vi "Import - Main.vi"(6 "New CD?":bool, 7 "Device Item Ref in":T19 format="%.0x", 8 "error in (no error)":errorcluster, 11 "Import/Export Data":T1 {"Tx Packets"."Tx Packet Data"."threadOptions"."pclDecimation" max=16 step=1; "Tx Packets"."Tx Packet Data"."threadOptions"."loopPeriod" max=16 step=1; "Tx Packets"."Tx Packet Data"."threadOptions"."targetPriority" min=-2 max=16 step=1; "Tx Packets"."Tx Packet Data"."threadOptions"."targetProcessor" min=-2 max=16 step=1; "Tx Packets"."Tx Packet Data"."Endianness" items=["big-endian"=0, "little-endian"=2]; "Rx Packets"."Rx Packet Data"."targetPriority" min=-2 max=16 step=1; "Rx Packets"."Rx Packet Data"."targetProcessor" min=-2 max=16 step=1; "Rx Packets"."Rx Packet Data"."Endianness" items=["big-endian"=0, "little-endian"=2]}) -> (0 "error out":errorcluster)   [LabVIEW 2019, in "UDP-Custom-Device System Explorer.lvlib"]
uses:
  UDP-Custom-Device System Explorer.lvlib
  <vilib>/NI VeriStand/Custom Device API/Custom Device Item Ref.ctl
  Types/XML - New/ImpExp - Data.ctl
  Types/XML - New/ImpExp - Main Data.ctl
  <vilib>/NI VeriStand/Custom Device API/Custom Device Item Info.ctl
  Types/XML - New/ImpExp - Rx Packets Data.ctl
  Types/XML - New/ImpExp - Rx Packet Data.ctl
  Shared/Types/Shared - Channel Data Type.ctl
  Shared/Types/Shared - Buffered.PacketInfo.ctl
  Shared/Types/Shared - Pointer Encoding.ctl
  Shared/Types/Shared - Receive Buffer Options.ctl
  Shared/Types/Shared - Transmit Buffer Options.ctl
  Shared/Types/Shared - New Data Options.ctl
  Shared/Types/Shared - Thread Management.ctl
  Types/XML - New/ImpExp - Tx Packets Data.ctl
  Types/XML - New/ImpExp - Tx Packet Data.ctl
  Shared/Types/Shared - Transmit Flag Options.ctl
  Shared/Types/Shared - Transmit Echo Options.ctl
  Types/Threading/Thread Configuration.ctl
  Types/Threading/Thread Sync Reference.ctl
  Property Accessors/Main Accessors.lvlib
  <vilib>/NI VeriStand/Custom Device API/Custom Device API.lvlib
  <vilib>/NI VeriStand/Custom Device Tools/Custom Device Utility Library/Custom Device Utility Library.lvlib
  Shared/UDP-Custom-Device Shared.lvlib
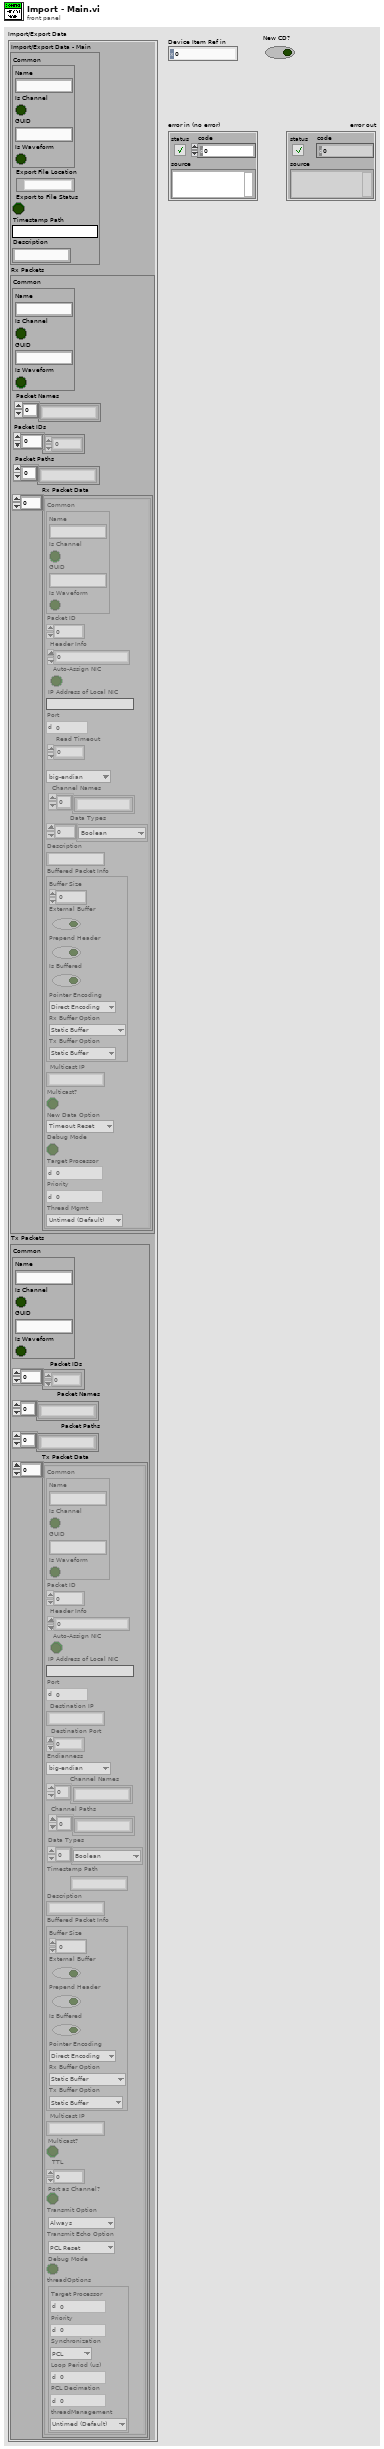
[diagram p1: front panel]
types:
  T1 = typedef "UDP-Custom-Device System Explorer.lvlib/ImpExp - Data.ctl" = cluster{"Import/Export Data - Main":T2, "Rx Packets":T4, "Tx Packets":T13}
  T2 = typedef "UDP-Custom-Device System Explorer.lvlib/ImpExp - Main Data.ctl" = cluster{"Common":T3, "Export File Location":path, "Export to File Status":bool, "Timestamp Path":string, "Description":string}
  T3 = typedef "Custom Device API.lvlib/Custom Device Item Info.ctl" = cluster{"Name":string, "Is Channel":bool, "GUID":string, "Is Waveform":bool}
  T4 = typedef "UDP-Custom-Device System Explorer.lvlib/ImpExp - Rx Packets Data.ctl" = cluster{"Common":T3, "Packet Names":string[], "Packet IDs":i32[], "Packet Paths":string[], "Rx Packet Data":T5[]}
  T5 = typedef "UDP-Custom-Device System Explorer.lvlib/ImpExp - Rx Packet Data.ctl" = cluster{"Common":T3, "Packet ID":i32, "Header Info":u32, "Auto-Assign NIC":bool, "IP Address of Local NIC":string, "Port":u16, "Read Timeout":i32, "Endianness":u16, "Channel Names":string[], "Data Types":T6[], "Description":string, "Buffered Packet Info":T7, "Multicast IP":string, "Multicast?":bool, "New Data Option":T11, "Debug Mode":bool, "targetProcessor":i8, "targetPriority":i16, "Thread Mgmt":T12}
  T6 = typedef "UDP-Custom-Device Shared.lvlib/Shared - Channel Data Type.ctl" = enum16{"Boolean", "Single", "Double", "I8", "I16", "I32", "I64", "U8", "U16", "U32", "U64"}
  T7 = typedef "UDP-Custom-Device Shared.lvlib/Shared - Buffered.PacketInfo.ctl" = cluster{"Buffer Size":i32, "External Buffer":bool, "Prepend Header":bool, "Is Buffered":bool, "Pointer Encoding":T8, "Rx Buffer Option":T9, "Tx Buffer Option":T10}
  T8 = typedef "UDP-Custom-Device Shared.lvlib/Shared - Pointer Encoding.ctl" = enum16{"Direct Encoding", "Conversion Encoding"}
  T9 = typedef "UDP-Custom-Device Shared.lvlib/Shared - Receive Buffer Options.ctl" = enum16{"Static Buffer", "Circular Buffer", "Circular Buffer + Size", "Internal Cache", "Internal Cache + Size", "Ping Pong", "Ping Pong + Size"}
  T10 = typedef "UDP-Custom-Device Shared.lvlib/Shared - Transmit Buffer Options.ctl" = enum16{"Static Buffer", "FIFO Buffer", "FIFO Buffer + Port"}
  T11 = typedef "UDP-Custom-Device Shared.lvlib/Shared - New Data Options.ctl" = enum16{"Timeout Reset", "Counter"}
  T12 = typedef "UDP-Custom-Device Shared.lvlib/Shared - Thread Management.ctl" = enum16{"Untimed (Default)", "Timed (High Priority)"}
  T13 = typedef "UDP-Custom-Device System Explorer.lvlib/ImpExp - Tx Packets Data.ctl" = cluster{"Common":T3, "Packet IDs":i32[], "Packet Names":string[], "Packet Paths":string[], "Tx Packet Data":T14[]}
  T14 = typedef "UDP-Custom-Device System Explorer.lvlib/ImpExp - Tx Packet Data.ctl" = cluster{"Common":T3, "Packet ID":i32, "Header Info":u32, "Auto-Assign NIC":bool, "IP Address of Local NIC":string, "Port":u16, "Destination IP":string, "Destination Port":u16, "Endianness":u16, "Channel Names":string[], "Channel Paths":string[], "Data Types":T6[], "Timestamp Path":string, "Description":string, "Buffered Packet Info":T7, "Multicast IP":string, "Multicast?":bool, "TTL":u16, "Port as Channel?":bool, "Transmit Option":T15, "Transmit Echo Option":T16, "Debug Mode":bool, "threadOptions":T17}
  T15 = typedef "UDP-Custom-Device Shared.lvlib/Shared - Transmit Flag Options.ctl" = enum16{"Always", "One-Shot", "Toggle"}
  T16 = typedef "UDP-Custom-Device Shared.lvlib/Shared - Transmit Echo Options.ctl" = enum16{"PCL Reset", "Counter", "Mirror"}
  T17 = typedef "UDP-Custom-Device System Explorer.lvlib/Thread Configuration.ctl" = cluster{"targetProcessor":i8, "targetPriority":i16, "Synchronization":T18, "loopPeriod":u32, "pclDecimation":u16, "threadManagement":T12}
  T18 = typedef "UDP-Custom-Device System Explorer.lvlib/Thread Sync Reference.ctl" = enum16{"PCL", "Async"}
  T19 = typedef "Custom Device API.lvlib/Custom Device Item Ref.ctl" = u64
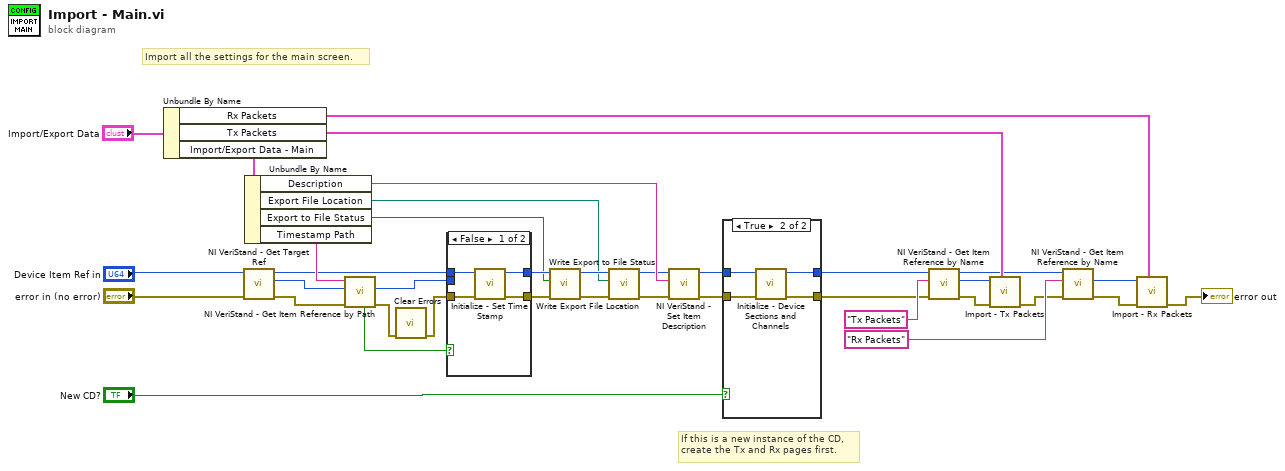
[diagram p0: block diagram]
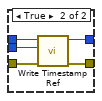
[diagram p2: hidden frame]
diagram:
  # "If this is a new instance of the CD,\ncreate the Tx and Rx pages first."
  # "Import all the settings for the main screen."
  n1 = Unbundle By Name("Import/Export Data") -> ("Rx Packets"=w17:T4, "Tx Packets"=w16:T13, "Import/Export Data - Main"=w36:T2)
  n2 = call <vilib>:"NI VeriStand - Get Target Ref.vi"("error in"="error in (no error)", "Item Ref in"="Device Item Ref in") -> ("error out"=w31:errorcluster, "Target Ref"=w33:T19, "Item Ref out"=w30:T19)  [unwired: 6 in, 1 out]
  n3 = Unbundle By Name(w36) -> ("Description"=w20:string, "Export File Location"=w21:path, "Export to File Status"=w22:bool, "Timestamp Path"=w35:string)
  n4 = call <vilib>:"NI VeriStand - Get Item Reference by Path.vi"("error in (no error)"=w31, "Root Ref"=w33, "Item Path in"=w35) -> ("error out"=w28:errorcluster, "Item Ref"=w29:T19, "Found"=w1:bool)  [unwired: 5 in, 1 out]
  n5 = call <vilib>:"Clear Errors.vi"("error in (no error)"=w28) -> ("error out"=w27:errorcluster)  [unwired: 5 in, 1 out]
  n6 = case shown="False" w1 {
    tunnel: w30 -> [w41 w46]
    tunnel: w29 -> [_ w45]
    tunnel: w27 -> [w39 w44]
    tunnel: [w40 w43] -> w26
    tunnel: [w38 w42] -> w25
    frame False {
      n7 = call "Initialize - Set Time Stamp.vi"("error in (no error)"=w39, "Device Item Ref in"=w41) -> ("error out"=w38:errorcluster, "Device Item Ref out"=w40:T19)  [unwired: 7 in, 1 out]
    }
    frame True {
      n8 = call "Write Timestamp Ref.vi"("error in (no error)"=w44, "Timestamp Ref"=w45, "Node Ptr"=w46) -> ("error out"=w42:errorcluster, "Node Ptr out"=w43:T19)  [unwired: 7 in]
    }
  }
  n9 = call "Write Export to File Status.vi"("error in (no error)"=w25, "Export to File Status"=w22, "Node Ptr"=w26) -> ("error out"=w24:errorcluster, "Node Ptr out"=w23:T19)  [unwired: 7 in]
  n10 = call "Write Export File Location.vi"("error in (no error)"=w24, "Export File Location"=w21, "Node Ptr"=w23) -> ("error out"=w18:errorcluster, "Node Ptr out"=w19:T19)  [unwired: 7 in]
  n11 = call <vilib>:"NI VeriStand - Set Item Description.vi"("error in (no error)"=w18, "Description"=w20, "Item Ref in"=w19) -> ("error out"=w13:errorcluster, "Item Ref out"=w15:T19)  [unwired: 6 in, 1 out]
  n12 = case shown="True" "New CD?" {
    tunnel: w15 -> [w48 w52]
    tunnel: w13 -> [w47 w51]
    tunnel: [w47 w50] -> w8
    tunnel: [w48 w49] -> w9
    frame False {
    }
    frame True {
      n13 = call "Initialize - Device Sections and Channels.vi"("error in (no error)"=w51, "Item Ref out"=w52) -> ("error out"=w50:errorcluster, "Parent Ref out"=w49:T19)  [unwired: 8 in]
    }
  }
  n14 = call <vilib>:"NI VeriStand - Get Item Reference by Name.vi"("error in (no error)"=w8, "Item Name"="Tx Packets" ("Section Name"), "Parent Ref in"=w9) -> ("error out"=w6:errorcluster, "Item Ref"=w7:T19, "Parent Ref out"=w12:T19)  [unwired: 5 in, 1 out]
  n15 = call "Import - Tx Packets.vi"("Tx Packets"=w16, "error in (no error)"=w6, "Device Item Ref in"=w7) -> ("error out"=w5:errorcluster)  [unwired: 8 in]
  n16 = call <vilib>:"NI VeriStand - Get Item Reference by Name.vi"("error in (no error)"=w5, "Item Name"="Rx Packets" ("Section Name"), "Parent Ref in"=w12) -> ("error out"=w3:errorcluster, "Item Ref"=w4:T19)  [unwired: 5 in, 2 out]
  n17 = call "Import - Rx Packets.vi"("Rx Packets"=w17, "error in (no error)"=w3, "Device Item Ref in"=w4) -> ("error out"=→"error out":errorcluster)  [unwired: 8 in]
